vi "Request Name.vi"(8 "error in (no error)":errorcluster, 10 "Name":string, 11 "LV Chat Client in":refnum<class "LV Chat Client.lvclass">) -> (0 "error out":errorcluster, 3 "LV Chat Client out":refnum<class "LV Chat Client.lvclass">)   [LabVIEW 2020, in "LV Chat Client.lvclass"]
uses:
  LV Chat Client.lvclass
  Data Types/User Info.ctl
  Data Types/Message ID.ctl
  LV Chat Client.lvclass/LV Chat Client.ctl
  fe732194-b45b-4a92-bcea-dea4a14a7d73.vi
  a534a8b3-ff78-4d94-b38a-4434f3f0a368.vi
  a534a8b3-ff78-4d94-b38a-4434f3f0a368.vi/43e93f4b-eb60-4448-b7e4-56a49cc750fb.vi
  a534a8b3-ff78-4d94-b38a-4434f3f0a368.vi/0bdc4188-3073-475f-bdb7-d424a9377977.vi
  Stream-Simple-Msg/Message/_Create.vi
  Stream-Simple-Msg/Manager/Get Endpoints.vi
  Stream-Simple-Msg/Message/Get Flattened Message.vi
  Stream-Simple-Msg/Endpoint/Get Stream.vi
  Stream-Simple-Msg/Message/Message.lvclass
  <vilib>/IlluminatedG/lv-stream/stream/Stream.lvclass
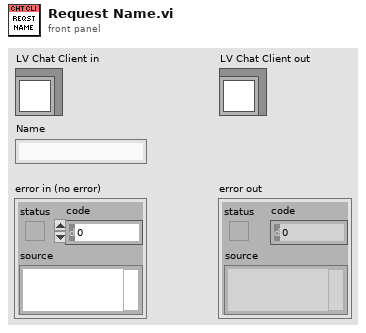
[diagram p1: front panel]
types:
  T1 = typedef "Message ID.ctl" = enum16{"UserInfo", "UserList", "Message", "Disconnect"}
  T2 = typedef "User Info.ctl" = cluster{"Name":string}
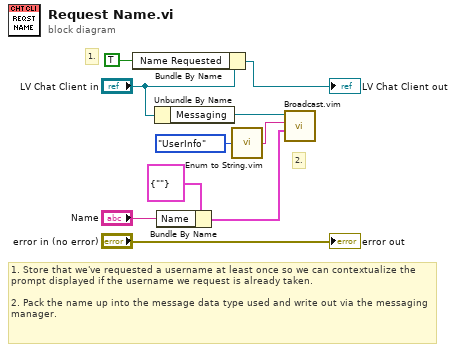
[diagram p0: block diagram]
diagram:
  # "1. Store that we've requested a username at least once so we can contextualize the prompt displayed if the username we request is already taken.\n\n2. Pack the name up into the message data type used and write out via the messaging manager."
  # "2."
  # "1."
  n1 = Bundle By Name(cluster="LV Chat Client in", "Name Requested"=TRUE ("Name Supplied")) -> (→"LV Chat Client out":refnum<class "LV Chat Client.lvclass">)
  n2 = Unbundle By Name("LV Chat Client in") -> ("Messaging"=w6:refnum<class "Manager.lvclass">)
  n3 = Bundle By Name(cluster=T2 {"Name"=""} ("User Info"), "Name"="Name") -> (w3:T2)
  n4 = call "Enum to String.vim"("Enum"=Message_ID."UserInfo" ("Message ID")) -> ("Enum String"=w1:string)
  n5 = call "Broadcast.vim"("Data (With ID String)"=w3, "Message (Or ID String)"=w1, "Manager in"=w6) -> ()  [unwired: 7 in, 2 out]
  "error out" <- "error in (no error)"
